vi "Чтение данных из Excel.vi"() -> ()   [LabVIEW 2018]
panel:
  in  "Выбор файла":path
  in  "Open":bool
  out "Загруженные данные:":string[][](table)=[["3", "FS10035937", "SP01E", "BB15", "MP56270101", "", "", "R", "", "", "", "", "", ""], ["4", "FS10035937", "SP01E", "BB16", "MP56270101", "", "", "R", "", "", "", "", "", ""], ["5", "", "SP02E", "1200", "MP56270101", "", "", "L", "", "", "", "", "", ""], ["6", "", "SP02E", "122", "MP56270101", "", "", "L", "", "", "", "", "", ""], ["7", "", "SP02E", "1220", "MP56270101", "", "", "L", "", "", "", "", "", ""]]
  in  "Array":string[][](array[string])
  in  "Загрузка Excel приложения":refnum<k7>
  in  "Excel._Worksheet 2":refnum<k7>
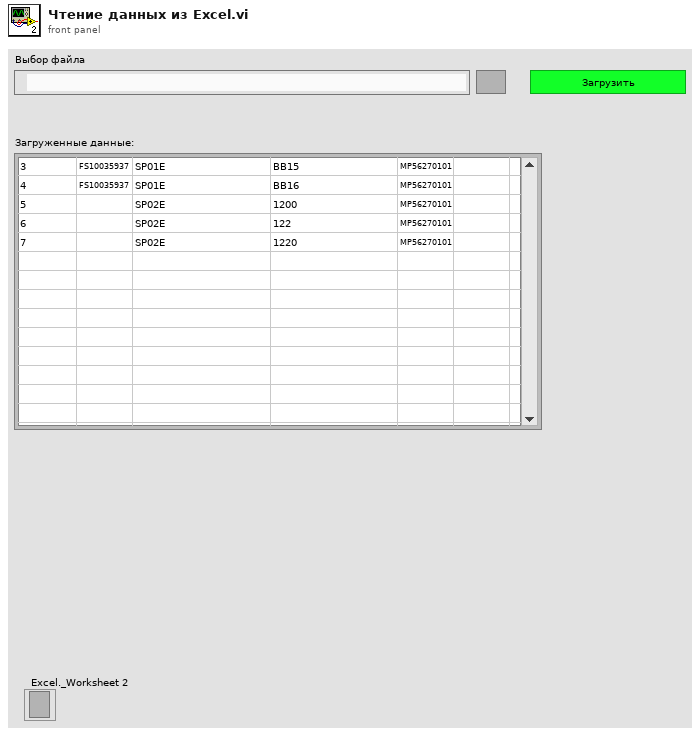
[diagram p1: front panel]
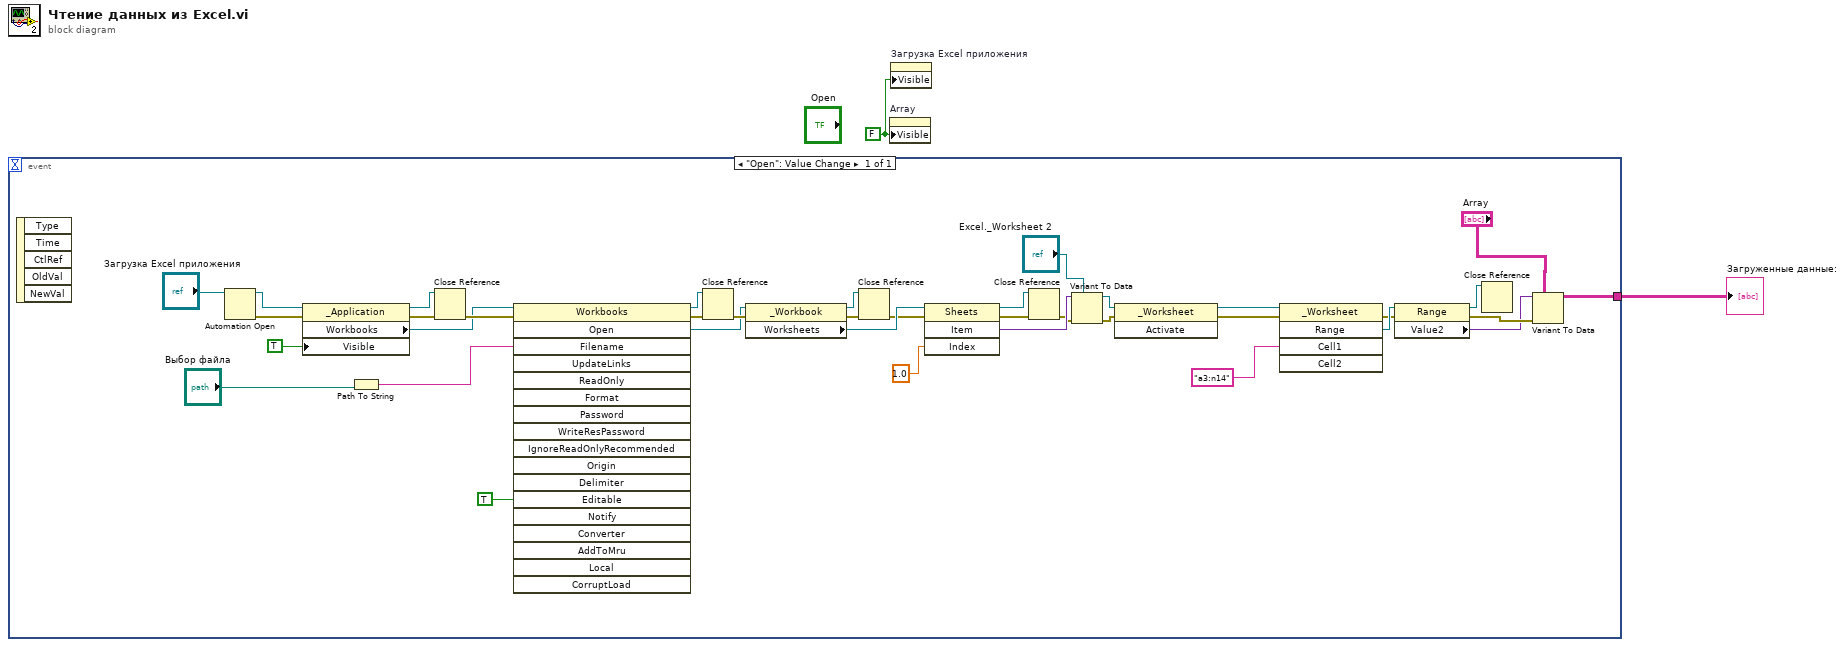
[diagram p0: block diagram]
diagram:
  w2 = FALSE ("Visible")
  n1 = event shown="[0] \"Open\": Value Change" {
    selector: _ -> [_]
    dyn-events: _ -> [_]
    timeout: _ -> [_]
    tunnel: [w6] -> w1
    event "Open": Value Change {
      n2 = event-data() -> ()  [unwired: 1 in, 5 out]
      n3 = Automation Open(Automation Refnum="Загрузка Excel приложения") -> (Automation Refnum=w39:refnum<k7>, error out=w26:errorcluster)  [unwired: 3 in]
      n4 = property class="_Application"(reference=w39, error in=w26, "Visible"=TRUE) -> (reference out=w24:refnum<k7>, error out=w19:errorcluster, "Workbooks"=w9:refnum<k7>)
      n5 = Path To String(path="Выбор файла") -> (string=w7:string)
      n6 = Close Reference(reference=w24, error in (no error)=w19) -> (error out=w18:errorcluster)
      n7 = invoke class="Workbooks" method="Open"(reference=w9, error in=w18, "Filename"=w7, "Editable"=TRUE) -> (reference out=w23:refnum<k7>, error out=w17:errorcluster, "Open"=w8:refnum<k7>)  [unwired: 14 in, 15 out]
      n8 = Close Reference(reference=w23, error in (no error)=w17) -> (error out=w16:errorcluster)
      n9 = property class="_Workbook"(reference=w8, error in=w16) -> (reference out=w22:refnum<k7>, error out=w15:errorcluster, "Worksheets"=w34:refnum<k7>)
      n10 = Close Reference(reference=w22, error in (no error)=w15) -> (error out=w14:errorcluster)
      n11 = invoke class="Sheets" method="Item"(reference=w34, error in=w14, "Index"=1.0) -> (reference out=w21:refnum<k7>, error out=w13:errorcluster, "Item"=w35:variant)  [unwired: 1 in, 1 out]
      n12 = Close Reference(reference=w21, error in (no error)=w13) -> (error out=w12:errorcluster)
      n13 = Variant To Data(error in=w12, type="Excel._Worksheet 2", Variant=w35) -> (data=w37:refnum<k7>, error out=w25:errorcluster)
      n14 = invoke class="_Worksheet" method="Activate"(reference=w37, error in=w25) -> (reference out=w28:refnum<k7>, error out=w11:errorcluster)  [unwired: 1 in, 1 out]
      n15 = invoke class="_Worksheet" method="Range"(reference=w28, error in=w11, "Cell1"="a3:n14") -> (error out=w10:errorcluster, "Range"=w30:refnum<k7>)  [unwired: 2 in, 3 out]
      n16 = property class="Range"(reference=w30, error in=w10) -> (reference out=w20:refnum<k7>, error out=w32:errorcluster, "Value2"=w31:variant)
      n17 = Close Reference(reference=w20) -> ()  [unwired: 1 in, 1 out]
      n18 = Variant To Data(error in=w32, type="Array", Variant=w31) -> (data=w6:string[][])  [unwired: 1 out]
    }
  }
  "Загруженные данные:" <- w1
  n19 = property on="Array" class="Arr (strict)"("Visible"=w2) -> ()  [unwired: 2 in, 2 out]
  n20 = property on="Загрузка Excel приложения" class="Ref (strict)"("Visible"=w2) -> ()  [unwired: 2 in, 2 out]
